vi "Open PowerSupply.vi"(8 "error in (no error)":errorcluster, 11 "PowerSupplyVisa-Fix in":refnum<class "PowerSupplyVisa-Fix.lvclass">) -> (0 "error out":errorcluster, 3 "PowerSupplyVisa-Fix out":refnum<class "PowerSupplyVisa-Fix.lvclass">)   [LabVIEW 2020, in "LAF2024Q2.lvlib" / "PowerSupplyVisa-Fix.lvclass"]
uses:
  PowerSupplyVisa-Fix.lvclass
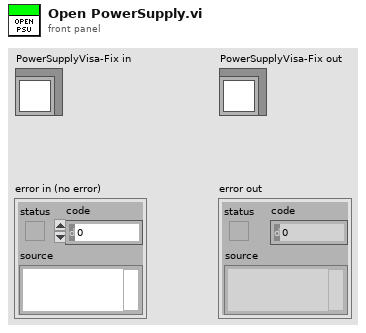
[diagram p1: front panel]
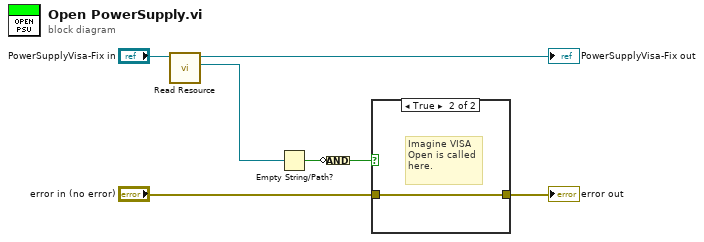
[diagram p0: block diagram]
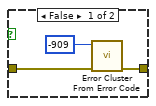
[diagram p2: hidden frame]
diagram:
  n1 = call-dynamic "Read Resource.vi"("PowerSupplyVisa-Fix in"="PowerSupplyVisa-Fix in") -> ("Resource"=w5:refnum<visa-resource-name>, "PowerSupplyVisa-Fix out"=→"PowerSupplyVisa-Fix out":refnum<class "PowerSupplyVisa-Fix.lvclass">)  [unwired: 8 in, 1 out]
  n2 = Empty String/Path?(string/path=w5) -> (empty?=w4:bool)
  n3 = Compound Arithmetic op=AND(invert w4) -> (w2:bool)
  n4 = case shown="True" w2 {
    tunnel: "error in (no error)" -> [w10 w11]
    tunnel: [w8 w11] -> w1
    frame False {
      n5 = call <vilib>:"Error Cluster From Error Code.vi"("error in (no error)"=w10, "error code (0)"=-909) -> ("error out"=w8:errorcluster)  [unwired: 7 in]
    }
    frame True {
      # "Imagine VISA Open is called here."
    }
  }
  "error out" <- w1
